vi "Export - Buffered Tx Packet.vi"(8 "error in (no error)":errorcluster, 11 "Device Item Ref in":T13 format="%.0x") -> (0 "error out":errorcluster, 3 "Tx Packet":T1 {"threadOptions"."pclDecimation" max=16 step=1; "threadOptions"."loopPeriod" max=16 step=1; "threadOptions"."targetPriority" min=-2 max=16 step=1; "threadOptions"."targetProcessor" min=-2 max=16 step=1; "Endianness" items=["big-endian"=0, "little-endian"=2]})   [LabVIEW 2019, in "UDP-Custom-Device System Explorer.lvlib"]
uses:
  UDP-Custom-Device System Explorer.lvlib
  <vilib>/NI VeriStand/Custom Device API/Custom Device Item Ref.ctl
  Types/XML - New/ImpExp - Tx Packet Data.ctl
  <vilib>/NI VeriStand/Custom Device API/Custom Device Item Info.ctl
  Shared/Types/Shared - Channel Data Type.ctl
  Shared/Types/Shared - Buffered.PacketInfo.ctl
  Shared/Types/Shared - Pointer Encoding.ctl
  Shared/Types/Shared - Receive Buffer Options.ctl
  Shared/Types/Shared - Transmit Buffer Options.ctl
  Shared/Types/Shared - Transmit Flag Options.ctl
  Shared/Types/Shared - Transmit Echo Options.ctl
  Types/Threading/Thread Configuration.ctl
  Types/Threading/Thread Sync Reference.ctl
  Shared/Types/Shared - Thread Management.ctl
  Property Accessors/Shared Packet Accessors.lvlib
  Property Accessors/Tx Packet Accessors.lvlib
  <vilib>/NI VeriStand/Custom Device API/Custom Device API.lvlib
  Shared/UDP-Custom-Device Shared.lvlib
  <vilib>/NI VeriStand/Custom Device Tools/Custom Device Utility Library/Custom Device Utility Library.lvlib
  Property Accessors/Buffered Data Packet.lvlib
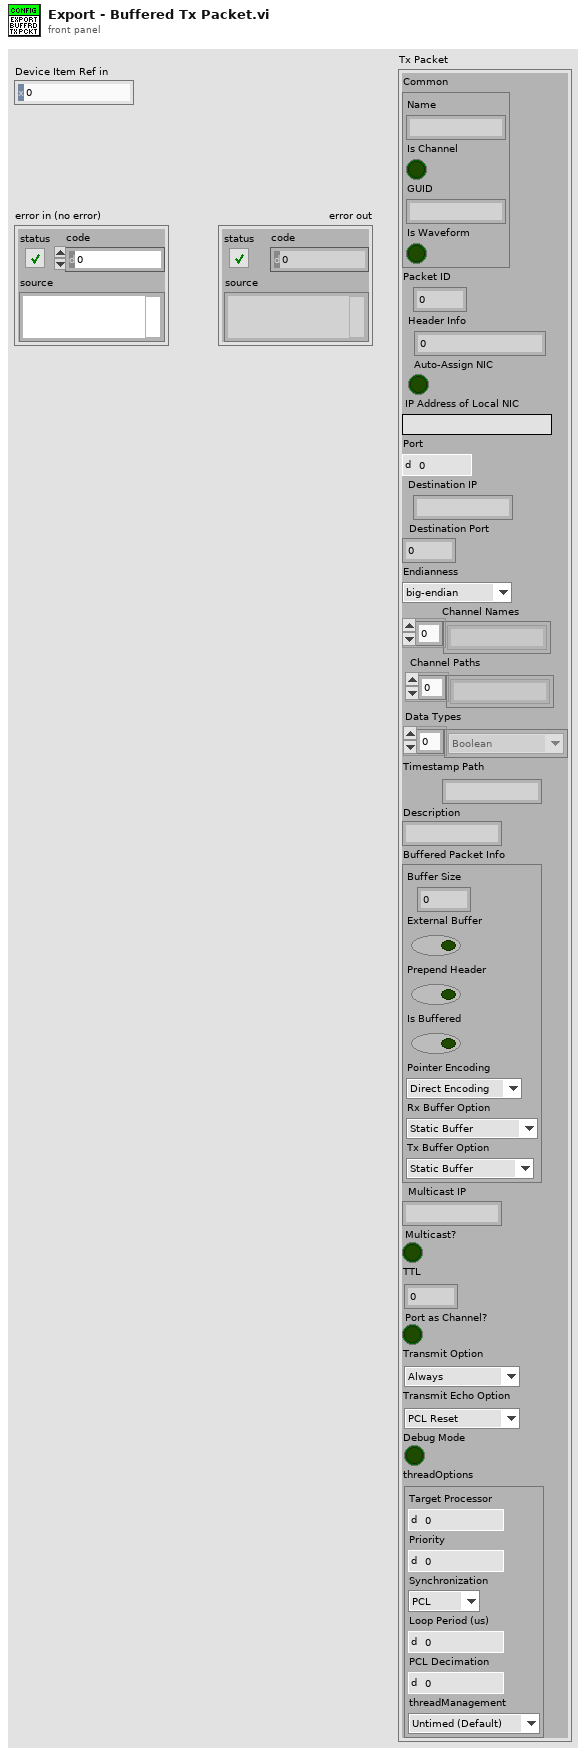
[diagram p1: front panel]
types:
  T1 = typedef "UDP-Custom-Device System Explorer.lvlib/ImpExp - Tx Packet Data.ctl" = cluster{"Common":T2, "Packet ID":i32, "Header Info":u32, "Auto-Assign NIC":bool, "IP Address of Local NIC":string, "Port":u16, "Destination IP":string, "Destination Port":u16, "Endianness":u16, "Channel Names":string[], "Channel Paths":string[], "Data Types":T3[], "Timestamp Path":string, "Description":string, "Buffered Packet Info":T4, "Multicast IP":string, "Multicast?":bool, "TTL":u16, "Port as Channel?":bool, "Transmit Option":T8, "Transmit Echo Option":T9, "Debug Mode":bool, "threadOptions":T10}
  T2 = typedef "Custom Device API.lvlib/Custom Device Item Info.ctl" = cluster{"Name":string, "Is Channel":bool, "GUID":string, "Is Waveform":bool}
  T3 = typedef "UDP-Custom-Device Shared.lvlib/Shared - Channel Data Type.ctl" = enum16{"Boolean", "Single", "Double", "I8", "I16", "I32", "I64", "U8", "U16", "U32", "U64"}
  T4 = typedef "UDP-Custom-Device Shared.lvlib/Shared - Buffered.PacketInfo.ctl" = cluster{"Buffer Size":i32, "External Buffer":bool, "Prepend Header":bool, "Is Buffered":bool, "Pointer Encoding":T5, "Rx Buffer Option":T6, "Tx Buffer Option":T7}
  T5 = typedef "UDP-Custom-Device Shared.lvlib/Shared - Pointer Encoding.ctl" = enum16{"Direct Encoding", "Conversion Encoding"}
  T6 = typedef "UDP-Custom-Device Shared.lvlib/Shared - Receive Buffer Options.ctl" = enum16{"Static Buffer", "Circular Buffer", "Circular Buffer + Size", "Internal Cache", "Internal Cache + Size", "Ping Pong", "Ping Pong + Size"}
  T7 = typedef "UDP-Custom-Device Shared.lvlib/Shared - Transmit Buffer Options.ctl" = enum16{"Static Buffer", "FIFO Buffer", "FIFO Buffer + Port"}
  T8 = typedef "UDP-Custom-Device Shared.lvlib/Shared - Transmit Flag Options.ctl" = enum16{"Always", "One-Shot", "Toggle"}
  T9 = typedef "UDP-Custom-Device Shared.lvlib/Shared - Transmit Echo Options.ctl" = enum16{"PCL Reset", "Counter", "Mirror"}
  T10 = typedef "UDP-Custom-Device System Explorer.lvlib/Thread Configuration.ctl" = cluster{"targetProcessor":i8, "targetPriority":i16, "Synchronization":T11, "loopPeriod":u32, "pclDecimation":u16, "threadManagement":T12}
  T11 = typedef "UDP-Custom-Device System Explorer.lvlib/Thread Sync Reference.ctl" = enum16{"PCL", "Async"}
  T12 = typedef "UDP-Custom-Device Shared.lvlib/Shared - Thread Management.ctl" = enum16{"Untimed (Default)", "Timed (High Priority)"}
  T13 = typedef "Custom Device API.lvlib/Custom Device Item Ref.ctl" = u64
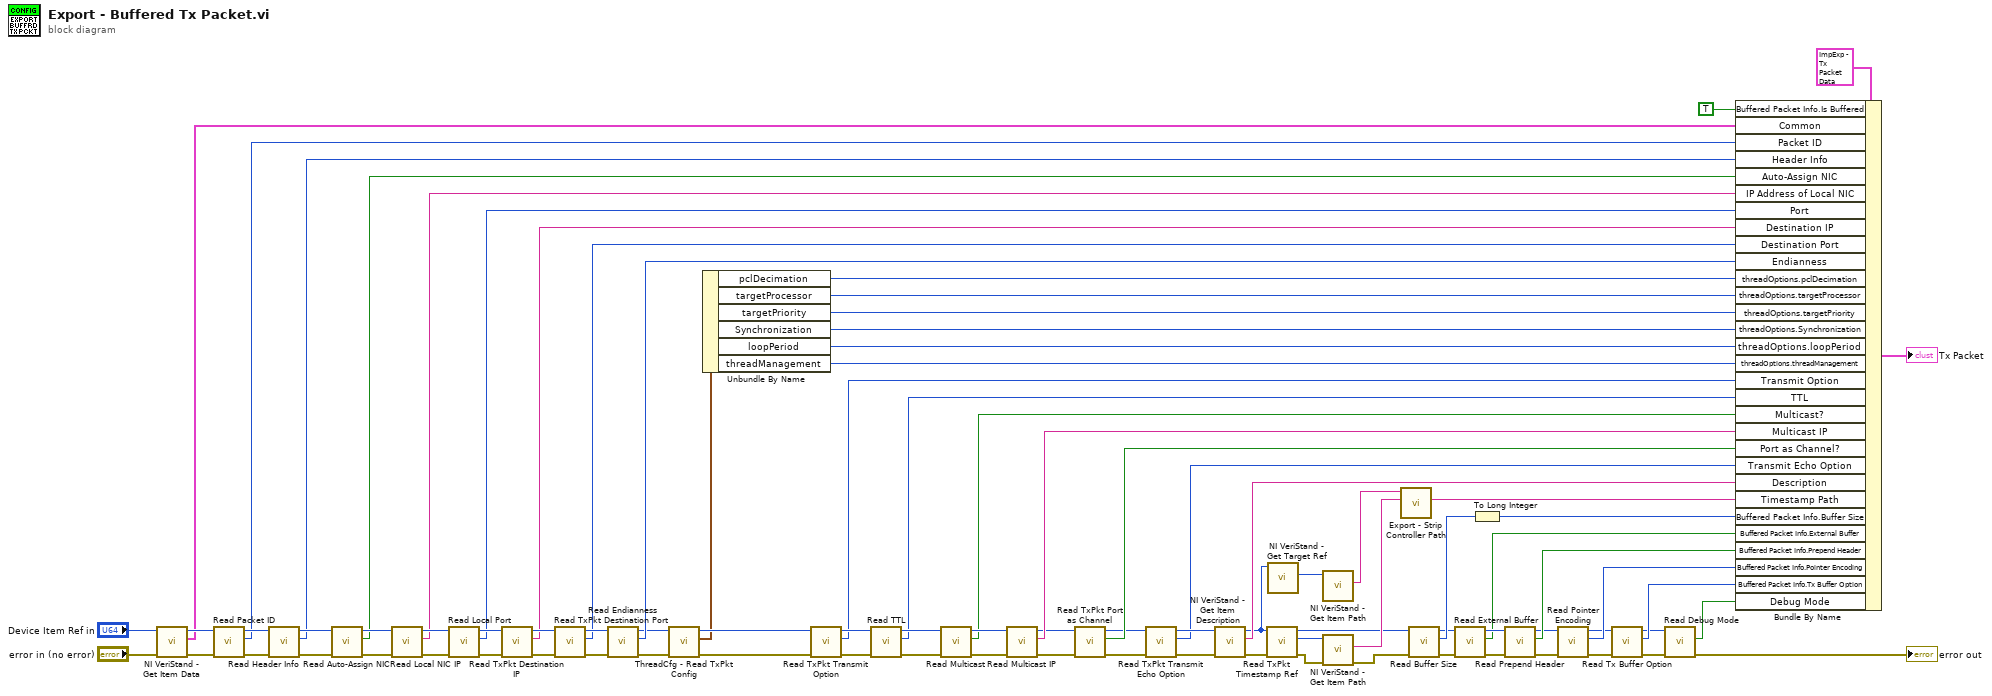
[diagram p0: block diagram]
diagram:
  n1 = call <vilib>:"NI VeriStand - Get Item Data.vi"("error in (no error)"="error in (no error)", "Item Ref in"="Device Item Ref in") -> ("error out"=w88:errorcluster, "Item Info"=w68:T2, "Item Ref out"=w73:T13)  [unwired: 6 in, 1 out]
  n2 = call "Read Packet ID.vi"("error in (no error)"=w88, "Node Ptr"=w73) -> ("error out"=w75:errorcluster, "Packet ID"=w67:i32, "Node Ptr out"=w74:T13)  [unwired: 7 in]
  n3 = call "Read Header Info.vi"("error in (no error)"=w75, "Node Ptr"=w74) -> ("error out"=w77:errorcluster, "Header Info"=w66:u32, "Node Ptr out"=w76:T13)  [unwired: 7 in]
  n4 = call "Read Auto-Assign NIC.vi"("error in (no error)"=w77, "Node Ptr"=w76) -> ("error out"=w81:errorcluster, "Auto-Assign NIC"=w65:bool, "Node Ptr out"=w78:T13)  [unwired: 7 in]
  n5 = call "Read Local NIC IP.vi"("error in (no error)"=w81, "Node Ptr"=w78) -> ("error out"=w80:errorcluster, "IP Address of Local NIC"=w64:string, "Node Ptr out"=w79:T13)  [unwired: 7 in]
  n6 = call "Read Local Port.vi"("error in (no error)"=w80, "Node Ptr"=w79) -> ("error out"=w83:errorcluster, "Port"=w63:u16, "Node Ptr out"=w82:T13)  [unwired: 7 in]
  n7 = call "Read TxPkt Destination IP.vi"("error in (no error)"=w83, "Node Ptr"=w82) -> ("error out"=w85:errorcluster, "Destination IP"=w62:string, "Node Ptr out"=w84:T13)  [unwired: 7 in]
  n8 = call "Read TxPkt Destination Port.vi"("error in (no error)"=w85, "Node Ptr"=w84) -> ("error out"=w87:errorcluster, "Destination Port"=w61:u16, "Node Ptr out"=w86:T13)  [unwired: 7 in]
  n9 = call "Read Endianness.vi"("error in (no error)"=w87, "Node Ptr"=w86) -> ("error out"=w9:errorcluster, "Endianness"=w60:u16, "Node Ptr out"=w11:T13)  [unwired: 7 in]
  n10 = call "ThreadCfg - Read TxPkt Config.vi"("error in (no error)"=w9, "Node Ptr In"=w11) -> ("error out"=w8:errorcluster, "threadOptions"=w7:T10, "Node Ptr Out"=w10:T13)  [unwired: 7 in]
  n11 = Unbundle By Name(w7) -> ("pclDecimation"=w6:u16, "targetProcessor"=w5:i8, "targetPriority"=w4:i16, "Synchronization"=w3:T11, "loopPeriod"=w2:u32, "threadManagement"=w1:T12)
  n12 = call "Read TxPkt Transmit Option.vi"("error in (no error)"=w8, "Node Ptr"=w10) -> ("error out"=w26:errorcluster, "Transmit Options"=w25:T8, "Node Ptr out"=w27:T13)  [unwired: 7 in]
  n13 = call "Read TTL.vi"("error in (no error)"=w26, "Node Ptr"=w27) -> ("error out"=w37:errorcluster, "TTL"=w36:u16, "Node Ptr out"=w40:T13)  [unwired: 7 in]
  n14 = call "Read Multicast.vi"("error in (no error)"=w37, "Node Ptr"=w40) -> ("error out"=w38:errorcluster, "Multicast"=w35:bool, "Node Ptr out"=w39:T13)  [unwired: 7 in]
  n15 = call "Read Multicast IP.vi"("error in (no error)"=w38, "Node Ptr"=w39) -> ("error out"=w29:errorcluster, "Multicast IP Address"=w34:string, "Node Ptr out"=w30:T13)  [unwired: 7 in]
  n16 = call "Read TxPkt Port as Channel.vi"("error in (no error)"=w29, "Node Ptr"=w30) -> ("error out"=w18:errorcluster, "Port as Channel"=w28:bool, "Node Ptr out"=w20:T13)  [unwired: 7 in]
  n17 = call "Read TxPkt Transmit Echo Option.vi"("error in (no error)"=w18, "Node Ptr"=w20) -> ("error out"=w17:errorcluster, "Transmit Echo Options"=w16:T9, "Node Ptr out"=w19:T13)  [unwired: 7 in]
  n18 = call <vilib>:"NI VeriStand - Get Item Description.vi"("error in (no error)"=w17, "Item Ref in"=w19) -> ("error out"=w56:errorcluster, "Description"=w59:string, "Item Ref out"=w52:T13)  [unwired: 6 in, 1 out]
  n19 = call "Read TxPkt Timestamp Ref.vi"("error in (no error)"=w56, "Node Ptr"=w52) -> ("error out"=w55:errorcluster, "Timestamp Ref"=w57:T13, "Node Ptr out"=w45:T13)  [unwired: 7 in]
  n20 = call <vilib>:"NI VeriStand - Get Target Ref.vi"("Item Ref in"=w52) -> ("Target Ref"=w53:T13)  [unwired: 7 in, 3 out]
  n21 = call <vilib>:"NI VeriStand - Get Item Path.vi"("Item Ref in"=w53) -> ("Path"=w51:string)  [unwired: 7 in, 3 out]
  n22 = call <vilib>:"NI VeriStand - Get Item Path.vi"("error in (no error)"=w55, "Item Ref in"=w57) -> ("error out"=w44:errorcluster, "Path"=w58:string)  [unwired: 6 in, 2 out]
  n23 = call "Export - Strip Controller Path.vi"("Channel Path"=w58, "Controller Path"=w51) -> ("Stripped Path"=w54:string)  [unwired: 8 in, 1 out]
  n24 = call "Read Buffer Size.vi"("error in (no error)"=w44, "Node Ptr"=w45) -> ("error out"=w48:errorcluster, "Buffer Size"=w50:u32, "Node Ptr out"=w46:T13)  [unwired: 7 in]
  n25 = call "Read External Buffer.vi"("error in (no error)"=w48, "Node Ptr"=w46) -> ("error out"=w49:errorcluster, "External Buffer"=w42:bool, "Node Ptr out"=w47:T13)  [unwired: 7 in]
  n26 = To Long Integer(number=w50) -> (32bit integer=w43:i32)
  n27 = call "Read Prepend Header.vi"("error in (no error)"=w49, "Node Ptr"=w47) -> ("error out"=w32:errorcluster, "Prepend Header"=w41:bool, "Node Ptr out"=w33:T13)  [unwired: 7 in]
  n28 = call "Read Pointer Encoding.vi"("error in (no error)"=w32, "Node Ptr"=w33) -> ("error out"=w23:errorcluster, "Pointer Encoding"=w31:T5, "Node Ptr out"=w24:T13)  [unwired: 7 in]
  n29 = call "Read Tx Buffer Option.vi"("error in (no error)"=w23, "Node Ptr"=w24) -> ("error out"=w14:errorcluster, "Buffer Option"=w22:T7, "Node Ptr out"=w15:T13)  [unwired: 7 in]
  n30 = call "Read Debug Mode.vi"("error in (no error)"=w14, "Node Ptr"=w15) -> ("error out"=→"error out":errorcluster, "Debug Mode"=w12:bool)  [unwired: 7 in, 1 out]
  n31 = Bundle By Name(cluster=T1 {"Common"={"Name"="", "Is Channel"=FALSE, "GUID"="", "Is Waveform"=FALSE}, "Packet ID"=0, "Header Info"=0, "Auto-Assign NIC"=FALSE, "IP Address of Local NIC"="", "Port"=0, "Destination IP"="", "Destination Port"=0, "Endianness"=0, "Channel Names"=[], "Channel Paths"=[], "Data Types"=[], "Timestamp Path"="", "Description"="", "Buffered Packet Info"={"Buffer Size"=0, "External Buffer"=FALSE, "Prepend Header"=FALSE, "Is Buffered"=FALSE, "Pointer Encoding"=enum."Direct Encoding", "Rx Buffer Option"=enum."Static Buffer", "Tx Buffer Option"=enum."Static Buffer"}, "Multicast IP"="", "Multicast?"=FALSE, "TTL"=0, "Port as Channel?"=FALSE, "Transmit Option"=enum."Always", "Transmit Echo Option"=enum."PCL Reset", "Debug Mode"=FALSE, "threadOptions"={"targetProcessor"=0, "targetPriority"=0, "Synchronization"=enum."PCL", "loopPeriod"=0, "pclDecimation"=0, "threadManagement"=enum."Untimed (Default)"}} ("Tx Packet"), "Buffered Packet Info.Is Buffered"=TRUE, "Common"=w68, "Packet ID"=w67, "Header Info"=w66, "Auto-Assign NIC"=w65, "IP Address of Local NIC"=w64, "Port"=w63, "Destination IP"=w62, "Destination Port"=w61, "Endianness"=w60, "threadOptions.pclDecimation"=w6, "threadOptions.targetProcessor"=w5, "threadOptions.targetPriority"=w4, "threadOptions.Synchronization"=w3, "threadOptions.loopPeriod"=w2, "threadOptions.threadManagement"=w1, "Transmit Option"=w25, "TTL"=w36, "Multicast?"=w35, "Multicast IP"=w34, "Port as Channel?"=w28, "Transmit Echo Option"=w16, "Description"=w59, "Timestamp Path"=w54, "Buffered Packet Info.Buffer Size"=w43, "Buffered Packet Info.External Buffer"=w42, "Buffered Packet Info.Prepend Header"=w41, "Buffered Packet Info.Pointer Encoding"=w31, "Buffered Packet Info.Tx Buffer Option"=w22, "Debug Mode"=w12) -> (→"Tx Packet":T1)
